vi "Link.vi"(0 "State in":refnum<class "State.lvclass">, 5 "Event Names":string[](array[string]), 7 "State Names":string[](array[string]), 11 "error in (no error)":errorcluster) -> (4 "State out":refnum<class "State.lvclass">, 15 "error out":errorcluster)   [LabVIEW 2020, in "State.lvclass"]
uses:
  State.lvclass
  State.lvclass/State.ctl
  Timeout/Timeout.lvclass
  Termination/Termination.lvclass
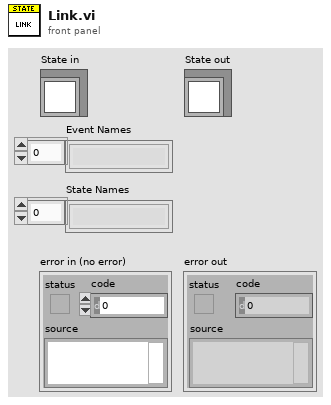
[diagram p1: front panel]
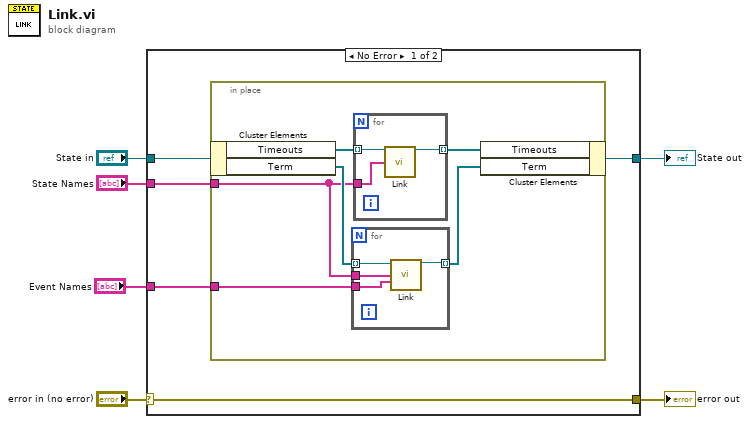
[diagram p0: block diagram]
diagram:
  n1 = case shown="No Error" "error in (no error)" {
    selector: "error in (no error)" -> [w11 w26]
    tunnel: [w11 w26] -> w5
    tunnel: [w9 w25] -> w3
    tunnel: "State in" -> [w10 w25]
    tunnel: "State Names" -> [w8 _]
    tunnel: "Event Names" -> [w7 _]
    frame No Error {
      n2 = in-place {
        in-place-border: w8 -> [w13]
        in-place-border: w7 -> [w12]
        n3 = in-place-cluster #1(w10) -> ("Timeouts"=w17:refnum<class "Timeout.lvclass">[], "Term"=w15:refnum<class "Termination.lvclass">[])
        n4 = for {
          tunnel: w15 -> [w24] mode=indexing
          tunnel: [w23] -> w14 mode=indexing
          tunnel: w13 -> [w22]
          tunnel: w12 -> [w21]
          n5 = call "Link.vi"("Termination in"=w24, "State names"=w22, "Event names"=w21) -> ("Termination out"=w23:refnum<class "Termination.lvclass">)  [unwired: 11 in, 1 out]
        }
        n6 = for {
          tunnel: w17 -> [w20] mode=indexing
          tunnel: [w19] -> w16 mode=indexing
          tunnel: w13 -> [w18]
          n7 = call "Link.vi"("Timeout in"=w20, "State names"=w18) -> ("Timeout out"=w19:refnum<class "Timeout.lvclass">)  [unwired: 12 in, 1 out]
        }
        n8 = in-place-cluster #1("Timeouts"=w16, "Term"=w14) -> (w9:refnum<class "State.lvclass">)
      }
    }
    frame Error {
    }
  }
  "error out" <- w5
  "State out" <- w3
